vi "fit histogram to exponential.vi"(8 "error in (no error)":errorcluster, 10 "num exp":i32=1, 11 "Y":dbl[](array[numeric])) -> (0 "error out":errorcluster, 1 "dead counts":dbl, 2 "exponential fit parameters":cluster{"t0":dbl, "amplitude":dbl}[](array[cluster]), 3 "best nonlinear fit":dbl[](array[numeric]), 4 "tau":dbl, 5 "initial guess":dbl[](array[numeric]))   [LabVIEW 2017]
uses:
  <vilib>/gmath/NumericalOptimization/Nonlinear Curve Fit LM bound.vi
  <vilib>/gmath/NI_Gmath.lvlib
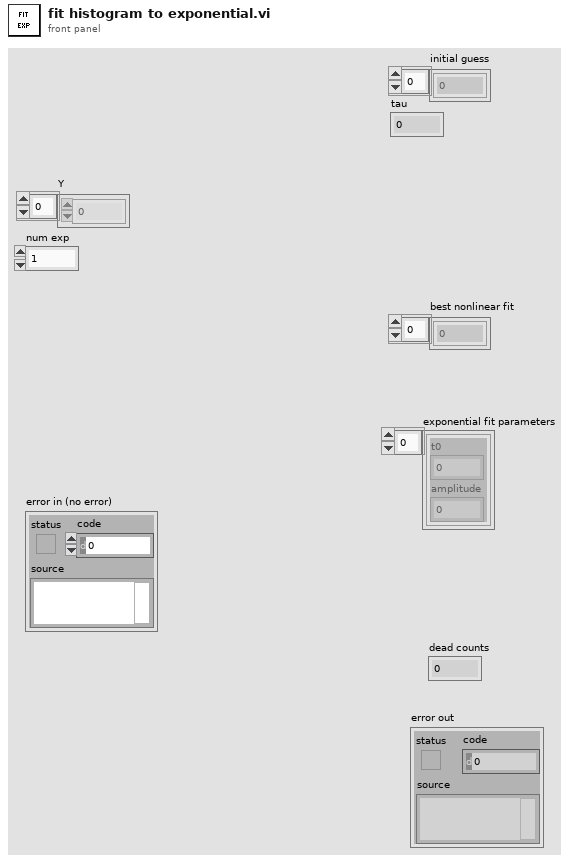
[diagram p1: front panel]
types:
  T1 = cluster{"parameter minimum":dbl[], "parameter maximum":dbl[]}
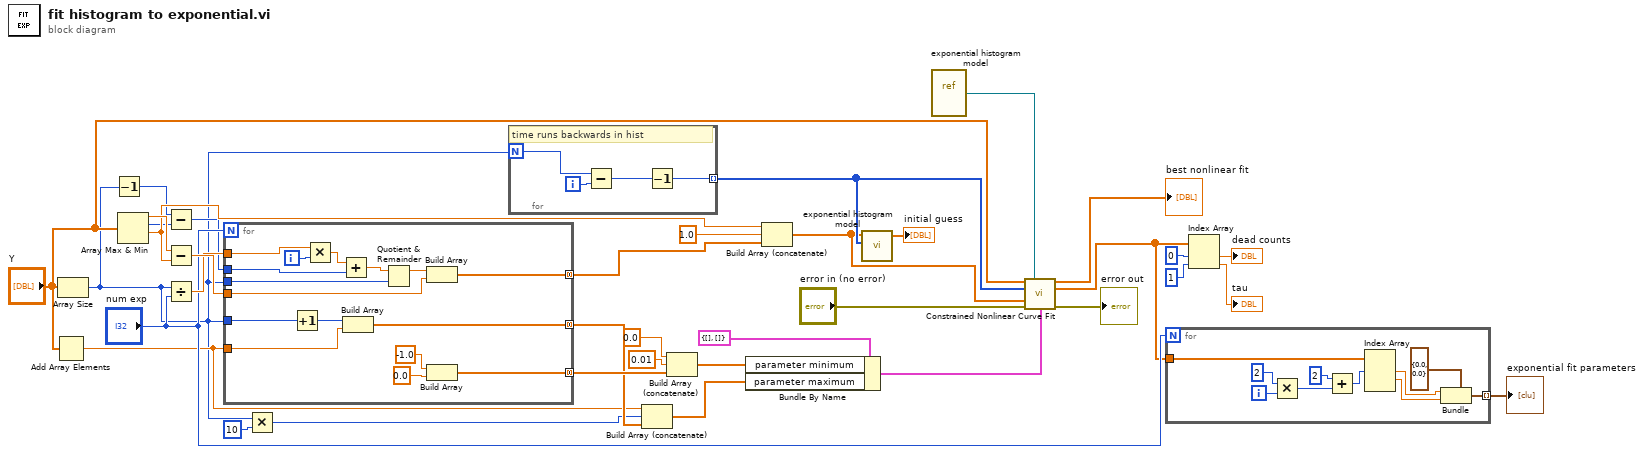
[diagram p0: block diagram]
diagram:
  n1 = Add Array Elements(numeric array="Y") -> (sum=w4:dbl)
  n2 = Array Size(array="Y") -> (size(s)=w3:i32)
  n3 = Decrement(x=w3) -> (x-1=w10:i32)
  n4 = Array Max & Min(array="Y") -> (max value=w36:dbl, max index (indices)=w12:i32, min value=w33:dbl)  [unwired: 1 out]
  n5 = Subtract(x=w10, y=w12) -> (x-y=w11:i32)
  n6 = Subtract(x=w36, y=w33) -> (x-y=w35:dbl)
  n7 = Divide(x=w3, y="num exp") -> (x/y=w34:dbl)
  n8 = for {
    N: "num exp" -> [_]
    tunnel: w35 -> [w52]
    tunnel: w34 -> [w51]
    tunnel: [w49] -> w9 mode=concatenating
    tunnel: [w46] -> w32 mode=concatenating
    tunnel: w3 -> [w45]
    tunnel: w4 -> [w44]
    tunnel: [w43] -> w30 mode=concatenating
    tunnel: w11 -> [w41]
    tunnel: w3 -> [w40]
    i -> [w50]
    n9 = Increment(x=w45) -> (x+1=w37:i32)
    n10 = Multiply(x=w51, y=w50) -> (x*y=w42:dbl)
    n11 = Add(x=w42, y=w41) -> (x+y=w39:dbl)
    n12 = Build Array(w37, w44) -> (w43:dbl[])
    n13 = Quotient & Remainder(x=w39, y=w40) -> (x-y*floor(x/y)=w38:dbl)  [unwired: 1 out]
    n14 = Build Array(w38, w52) -> (w49:dbl[])
    n15 = Build Array(-1.0 ("element"), 0.0 ("element")) -> (w46:dbl[])
  }
  n16 = Multiply(x=w3, y=10) -> (x*y=w1:i32)
  n17 = for {
    N: w3 -> [w56]
    tunnel: [w53] -> w15 mode=indexing
    i -> [w55]
    # "time runs backwards in hist"
    n18 = Subtract(x=w56, y=w55) -> (x-y=w54:i32)
    n19 = Decrement(x=w54) -> (x-1=w53:i32)
  }
  n20 = Build Array (concatenate)(w4, w1, w30) -> (w27:dbl[])
  n21 = Build Array (concatenate)(0.0 ("element"), 0.01 ("element"), w32) -> (w28:dbl[])
  n22 = Bundle By Name(cluster=T1 {"parameter minimum"=[], "parameter maximum"=[]} ("parameter bounds"), "parameter minimum"=w28, "parameter maximum"=w27) -> (w26:T1)
  n23 = Build Array (concatenate)(w33, 1.0, w9) -> (w14:dbl[])
  n24 = call "exponential histogram model.vi"("X"=w15, "a"=w14) -> ("f(X,a)"=→"initial guess":dbl[])  [unwired: 2 in, 2 out]
  n25 = vi-ref "exponential histogram model.vi"() -> (w19:refnum<vi>)
  n26 = call-poly <vilib>:"Constrained Nonlinear Curve Fit.vi"("Y"="Y", "f(x,a)"=w19, "X"=w15, "initial parameters"=w14, "error in (no error)"="error in (no error)", "parameter bounds"=w26) -> ("best nonlinear fit"=→"best nonlinear fit":dbl[], "best fit parameters"=w23:dbl[], "error out"=→"error out":errorcluster)  [unwired: 4 in, 3 out]
  n27 = for {
    N: "num exp" -> [_]
    tunnel: w23 -> [w63]
    tunnel: [w59] -> w24 mode=indexing
    i -> [w66]
    n28 = Multiply(x=2, y=w66) -> (x*y=w65:i32)
    n29 = Add(x=2, y=w65) -> (x+y=w62:i32)
    n30 = Index Array(array=w63, index #1=w62) -> (element #1=w61:dbl, element #2=w60:dbl)  [unwired: 2 in, 1 out]
    n31 = Bundle(cluster=cluster{"t0":dbl, "amplitude":dbl} {"t0"=0.0, "amplitude"=0.0} ("Cluster"), "t0"=w61, "amplitude"=w60) -> (w59:cluster{"t0":dbl, "amplitude":dbl})
  }
  "exponential fit parameters" <- w24
  n32 = Index Array(array=w23, index #1=0 ("index"), index #2=1 ("index")) -> (element #1=→"dead counts":dbl, element #2=→"tau":dbl)
